vi "HoloPy_calc_mean_image.vi"(6 "imageSize":cluster{"image_size_X":i32, "image_size_Y":i32}, 8 "error in (no error)":errorcluster, 9 "imageFileExtension":string, 10 "directory path":path, 11 "Refnum in":refnum<k35>) -> (0 "error out":errorcluster, 2 "Array":sgl[][](array[numeric]), 3 "Refnum out":refnum<k35>)   [LabVIEW 2023, in "holoPyTracks.lvlib"]
uses:
  holoPyTracks.lvlib
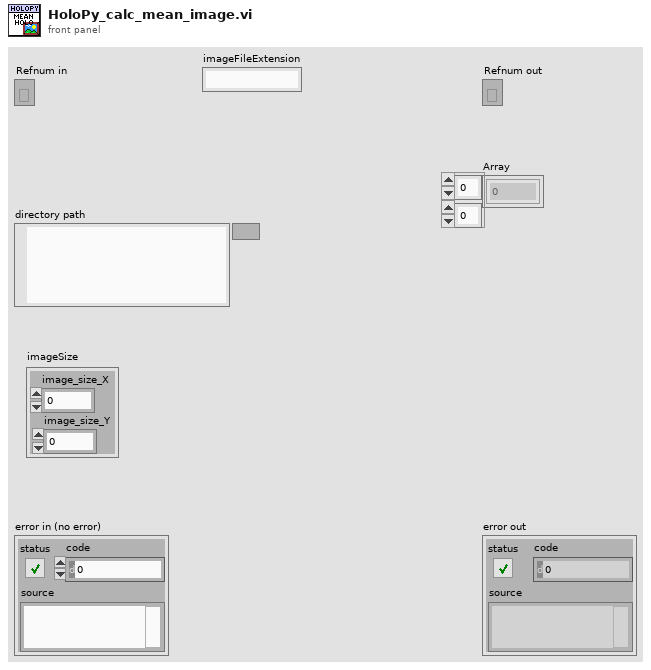
[diagram p1: front panel]
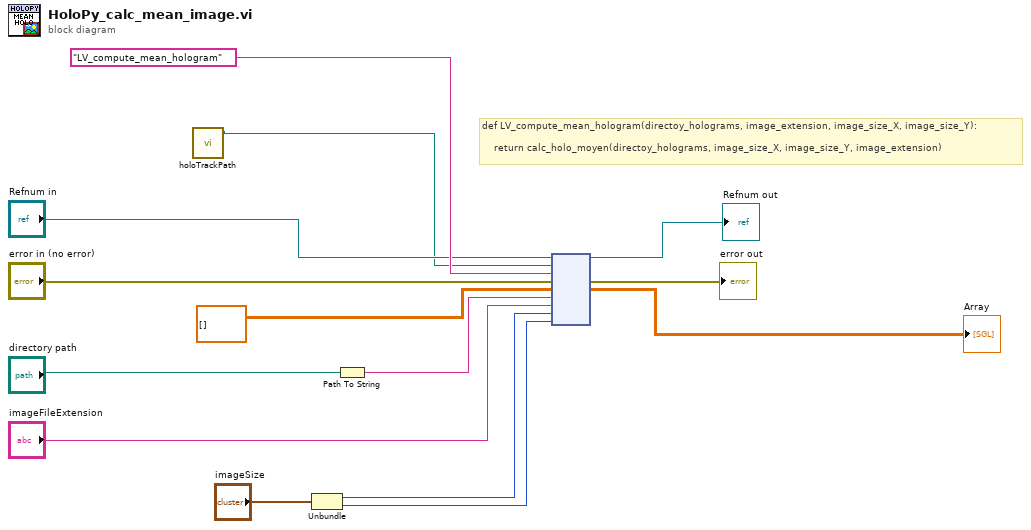
[diagram p0: block diagram]
diagram:
  # "def LV_compute_mean_hologram(directoy_holograms, image_extension, image_size_X, image_size_Y):\n\n    return calc_holo_moyen(directoy_holograms, image_size_X, image_size_Y, image_extension)"
  n1 = call "holoTrackPath.vi"() -> ("appended path"=w1:path)  [unwired: 11 in]
  n2 = Unbundle("imageSize") -> ("image_size_X"=w3:i32, "image_size_Y"=w2:i32)
  n3 = Path To String(path="directory path") -> (string=w14:string)
  n4 = node("Refnum in", w1, "LV_compute_mean_hologram" ("function name"), "error in (no error)", sgl[][] [], w14, "imageFileExtension", w3, w2) -> (→"Refnum out":refnum<k35>, →"error out":errorcluster, →"Array":sgl[][])  [unwired: 4 in, 2 out]
